vi "Core Write DAQ FIFO.vi"(6 "FIFO Timestamps":T2, 8 "error in (no error)":errorcluster, 9 "Timeout (ms)":i32=100, 10 "DAQ In":T1[](array[typedef]), 11 "CIFTag in":refnum<class "CIF_NIChn_Fifo_DAQ.lvclass">) -> (0 "error out":errorcluster, 1 "timed out?":bool, 2 "DAQ Out":T1[](array[typedef]), 3 "CIFTag out":refnum<class "CIF_NIChn_Fifo_DAQ.lvclass">)   [LabVIEW 2021, in "CIF_NIChn_Fifo_DAQ.lvclass"]
uses:
  CIF_NIChn_Fifo_DAQ.lvclass
  ChannelCommon/typedef/TimeStamps.ctl
  ChannelCommon/typedef/Datatype Waveform.ctl
  CIF_NIChn_Fifo_DAQ.lvclass/CIF_NIChn_Fifo_DAQ.ctl
  ChannelCommon/ChannelCommon.lvlib
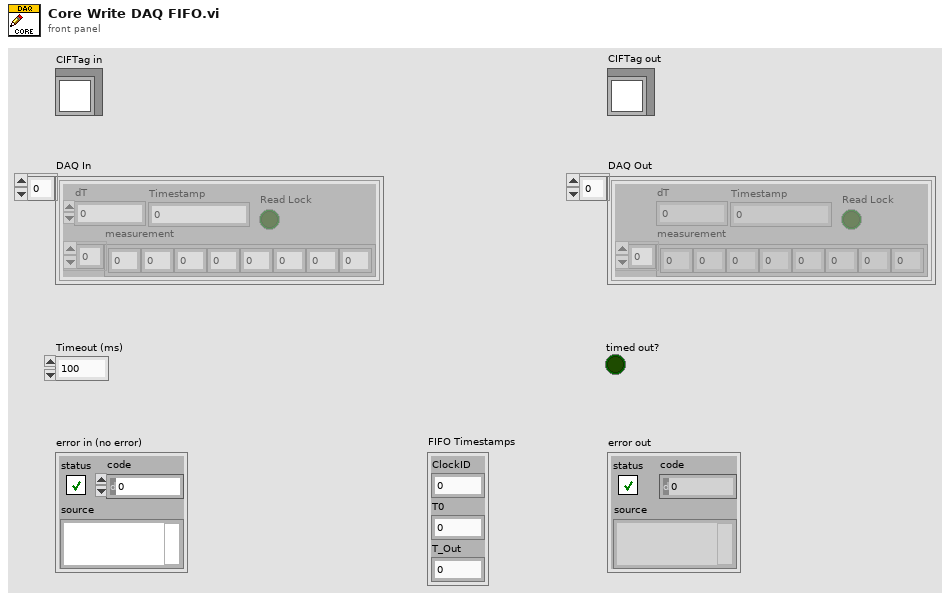
[diagram p1: front panel]
types:
  T1 = typedef "ChannelCommon.lvlib/Datatype Waveform.ctl" = cluster{"measurement":dbl[], "dT":dbl, "Timestamp":u64, "Read Lock":bool}
  T2 = typedef "ChannelCommon.lvlib/TimeStamps.ctl" = cluster{"ClockID":u8, "T0":i64, "T_Out":i64}
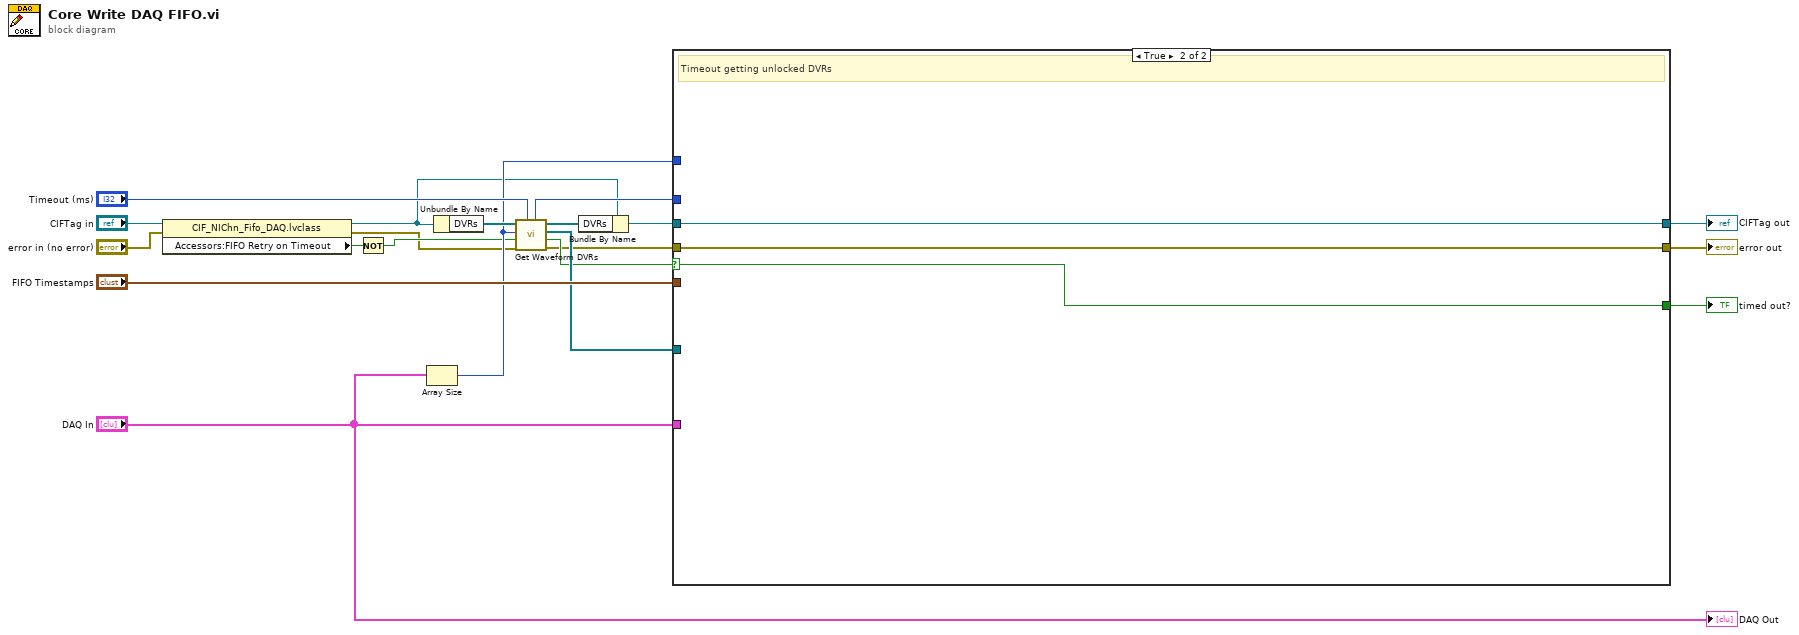
[diagram p0: block diagram]
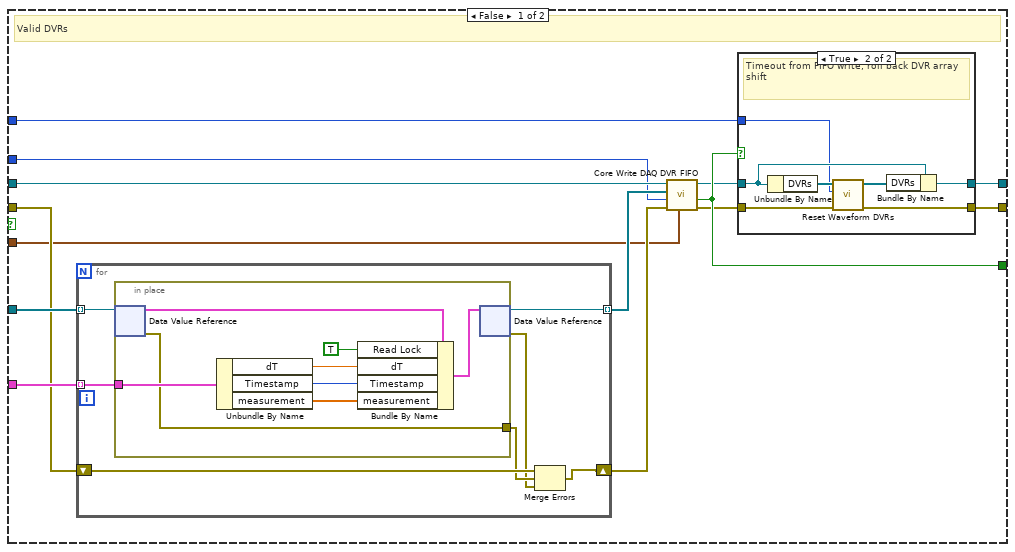
[diagram p2: hidden frame]
diagram:
  n1 = property class="CIF_NIChn_Fifo_DAQ.lvclass"(reference="CIFTag in", error in="error in (no error)") -> (reference out=w3:refnum<class "CIF_NIChn_Fifo_DAQ.lvclass">, error out=w1:errorcluster, "Accessors:FIFO Retry on Timeout"=w5:bool)
  n2 = Not(x=w5) -> (.not. x?=w2:bool)
  n3 = Array Size(array="DAQ In") -> (size(s)=w7:i32)
  n4 = Unbundle By Name(w3) -> ("DVRs"=w16:refnum<data-value>[])
  n5 = call "Get Waveform DVRs.vi"("Timeout in (ms)"="Timeout (ms)", "error in (no error)"=w1, "Ignore Read Lock"=w2, "Number of Waveforms"=w7, "DVR Circular Buffer in"=w16) -> ("error out"=w10:errorcluster, "Timeout"=w11:bool, "DVRs"=w12:refnum<data-value>[], "DVR Circular Buffer out"=w15:refnum<data-value>[], "Remaining timeout (ms)"=w9:i32)  [unwired: 2 in]
  n6 = Bundle By Name(cluster=w3, "DVRs"=w15) -> (w13:refnum<class "CIF_NIChn_Fifo_DAQ.lvclass">)
  n7 = case shown="True" w11 {
    selector: w11 -> [_ w59]
    tunnel: w10 -> [w31 w60]
    tunnel: w13 -> [w34 w61]
    tunnel: w12 -> [w33 _]
    tunnel: [w24 w61] -> w20
    tunnel: [w26 w59] -> w19
    tunnel: [w22 w60] -> w18
    tunnel: "DAQ In" -> [w32 _]
    tunnel: "FIFO Timestamps" -> [w28 _]
    tunnel: w9 -> [w27 _]
    tunnel: w7 -> [w21 _]
    frame False {
      # "Valid DVRs"
      n8 = for {
        tunnel: w33 -> [w50] mode=indexing
        tunnel: w32 -> [w49] mode=indexing
        tunnel: [w48] -> w29 mode=indexing
        shift-right: [w44] -> w30
        shift-left: w31 -> [w47]
        n9 = in-place {
          in-place-border: w49 -> [w55]
          in-place-border: [w53] -> w46
          n10 = in-place-dvr #1(w50) -> (w58:T1, w53:errorcluster)
          n11 = Unbundle By Name(w55) -> ("dT"=w57:dbl, "Timestamp"=w56:u64, "measurement"=w51:dbl[])
          n12 = Bundle By Name(cluster=w58, "Read Lock"=TRUE, "dT"=w57, "Timestamp"=w56, "measurement"=w51) -> (w54:T1)
          n13 = in-place-dvr #1(w54) -> (w48:refnum<data-value>, w45:errorcluster)
        }
        n14 = Merge Errors(w47, w46, w45) -> (w44:errorcluster)
      }
      n15 = call "Core Write DAQ DVR FIFO.vi"("FIFO Timestamps"=w28, "error in (no error)"=w30, "Timeout (ms)"=w27, "Data In"=w29, "CIFTag in"=w34) -> ("error out"=w23:errorcluster, "timed out?"=w26:bool, "CIFTag out"=w25:refnum<class "CIF_NIChn_Fifo_DAQ.lvclass">)  [unwired: 3 in, 1 out]
      n16 = case shown="True" w26 {
        tunnel: w25 -> [w36 w43]
        tunnel: [w36 w42] -> w24
        tunnel: w23 -> [w35 w41]
        tunnel: [w35 w40] -> w22
        tunnel: w21 -> [_ w37]
        frame False {
        }
        frame True {
          # "Timeout from FIFO write, roll back DVR array shift"
          n17 = Unbundle By Name(w43) -> ("DVRs"=w38:refnum<data-value>[])
          n18 = call "Reset Waveform DVRs.vi"("error in (no error)"=w41, "Number of Waveforms"=w37, "DVR Circular Buffer in"=w38) -> ("error out"=w40:errorcluster, "DVR Circular Buffer out"=w39:refnum<data-value>[])  [unwired: 7 in]
          n19 = Bundle By Name(cluster=w43, "DVRs"=w39) -> (w42:refnum<class "CIF_NIChn_Fifo_DAQ.lvclass">)
        }
      }
    }
    frame True {
      # "Timeout getting unlocked DVRs"
    }
  }
  "error out" <- w18
  "CIFTag out" <- w20
  "timed out?" <- w19
  "DAQ Out" <- "DAQ In"
